vi "Enable.vi"(8 "error in (no error)":errorcluster, 9 "Chan":i32, 10 "Enable":bool, 11 "reference in":refnum<class "PSU_Keysight_34951A.lvclass">) -> (0 "error out":errorcluster, 3 "reference in":refnum<class "PSU_Keysight_34951A.lvclass">)   [LabVIEW 2022 SP3, in "PSU_Keysight_34951A.lvlib" / "PSU_Keysight_34951A.lvclass"]
uses:
  PSU_Keysight_34951A.lvclass
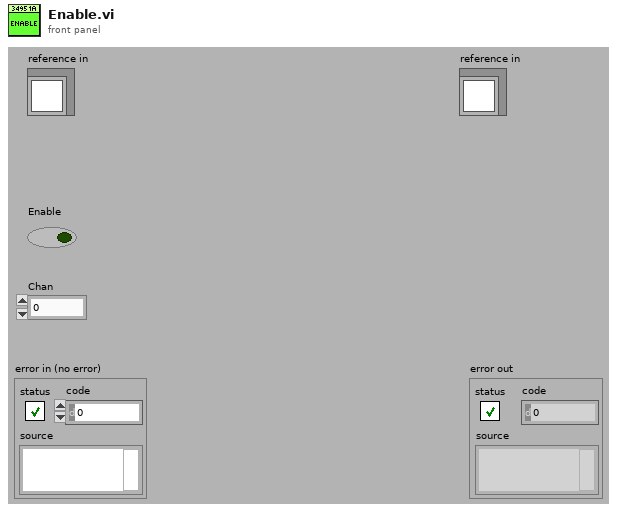
[diagram p1: front panel]
types:
  T1 = typedef "PSU_Keysight_34951A.lvlib/PSU_Keysight_34951A.lvclass/ObjectAttributes.ctl" = cluster{"Config":T2, "VISA res":refnum<visa-resource-name>, "Enabled":bool[], "V":dbl[], "I":dbl[], "Source Type":enum16{"Voltage", "Current"}[]}
  T2 = typedef "PSU_Keysight_34951A.lvlib/PSU_Keysight_34951A.lvclass/Config.ctl" = cluster{"VISA":refnum<visa-resource-name>, "Slot":i32}
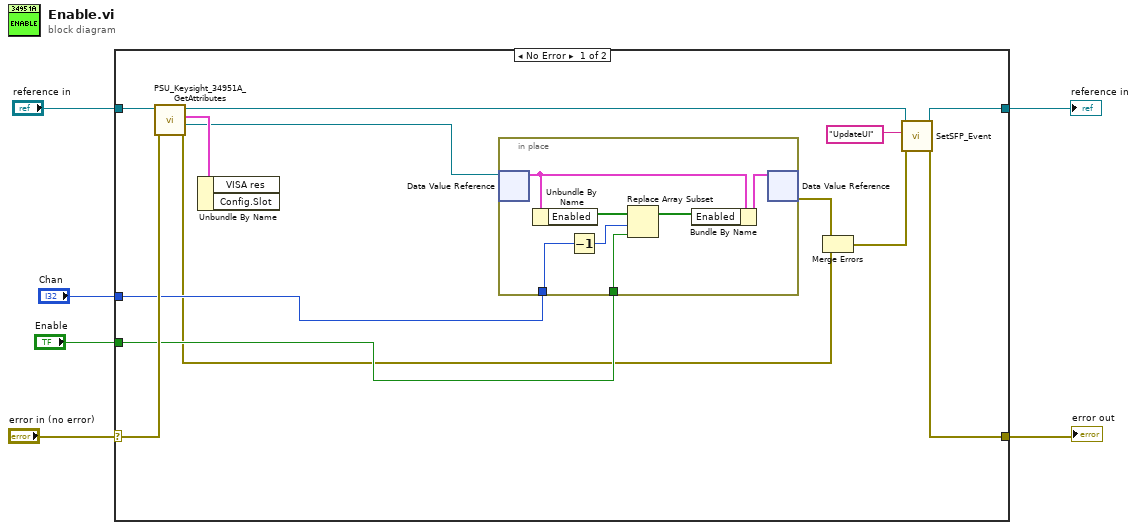
[diagram p0: block diagram]
diagram:
  n1 = case shown="No Error" "error in (no error)" {
    selector: "error in (no error)" -> [w19 w28]
    tunnel: [w14 w28] -> w5
    tunnel: [w9 w27] -> w3
    tunnel: "reference in" -> [w17 w27]
    tunnel: "Enable" -> [w12 _]
    tunnel: "Chan" -> [w13 _]
    frame No Error {
      n2 = call "PSU_Keysight_34951A_GetAttributes.vi"("error in (no error)"=w19, "reference in"=w17) -> ("error out"=w7:errorcluster, "DataRef"=w11:refnum<data-value>, "Data"=w18:T1, "reference out"=w10:refnum<class "PSU_Keysight_34951A.lvclass">)  [unwired: 6 in]
      n3 = Unbundle By Name(w18) -> ()  [unwired: 2 out]
      n4 = in-place {
        in-place-border: w13 -> [w24]
        in-place-border: w12 -> [w20]
        n5 = in-place-dvr #1(w11) -> (w25:T1)  [unwired: 1 out]
        n6 = Unbundle By Name(w25) -> ("Enabled"=w23:bool[])
        n7 = Decrement(x=w24) -> (x-1=w21:i32)
        n8 = Replace Array Subset(array=w23, new element=w20, index=w21) -> (w22:bool[])
        n9 = Bundle By Name(cluster=w25, "Enabled"=w22) -> (w26:T1)
        n10 = in-place-dvr #1(w26) -> (w16:errorcluster)  [unwired: 1 out]
      }
      n11 = Merge Errors(w16, w7) -> (w15:errorcluster)
      n12 = call-dynamic "SetSFP_Event.vi"("error in (no error)"=w15, "msg"="UpdateUI" ("Ancestor"), "reference in"=w10) -> ("error out"=w14:errorcluster, "reference out"=w9:refnum<class "PSU_Keysight_34951A.lvclass">)  [unwired: 7 in]
    }
    frame Error {
    }
  }
  "error out" <- w5
  "reference in" <- w3
